vi "Read Digital Transition Type.vi"(9 "Plot in":refnum<class "Plot.lvclass">) -> (3 "Plot out":refnum<class "Plot.lvclass">, 4 "Digital Transition Type":u8)   [LabVIEW 2014, in "Plot.lvclass"]
uses:
  Plot.lvclass
  Plot.lvclass/Plot.ctl
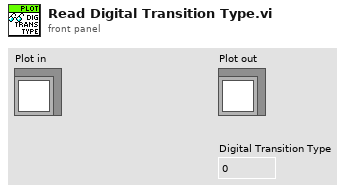
[diagram p1: front panel]
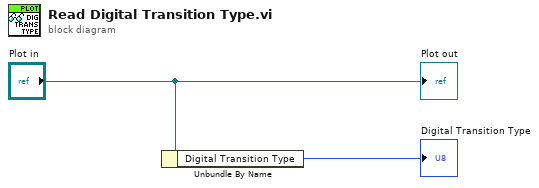
[diagram p0: block diagram]
diagram:
  n1 = Unbundle By Name("Plot in") -> ("Digital Transition Type"=→"Digital Transition Type":u8)
  "Plot out" <- "Plot in"
